vi "roboRIO Update Name Color.vi"(7 "FcdVI Ref":refnum<vi>, 8 "error in (no error)":errorcluster, 11 "Connector Name Ref":refnum<vi>) -> (0 "error out":errorcluster)   [LabVIEW 2021]
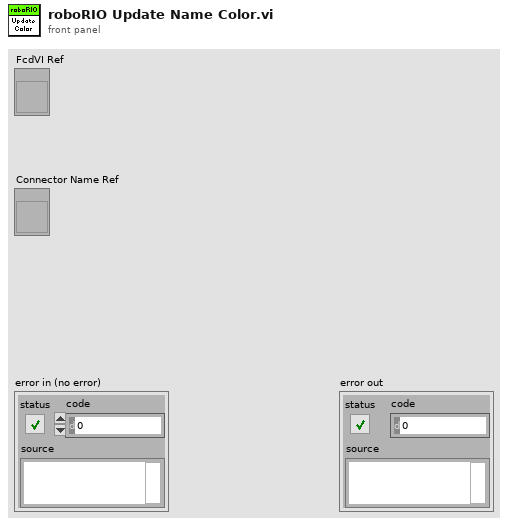
[diagram p1: front panel]
types:
  T1 = typedef "LVForegroundBackgroundColorsTypeDef.ctl" = cluster{"FG Color":u32, "BG Color":u32}
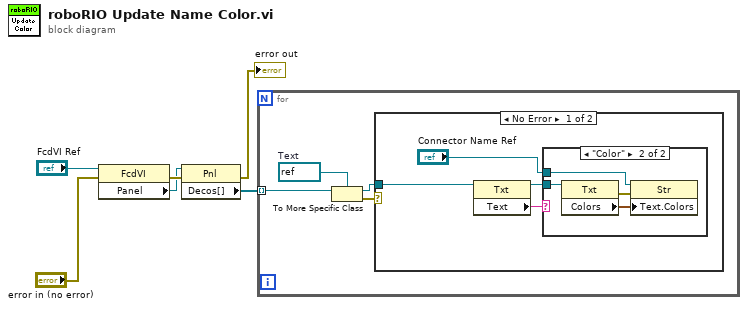
[diagram p0: block diagram]
diagram:
  n1 = property class="FcdVI"(reference="FcdVI Ref", error in="error in (no error)") -> (error out=w5:errorcluster, "Panel"=w4:refnum<vi>)  [unwired: 1 out]
  n2 = property class="Pnl"(reference=w4, error in=w5) -> (error out=→"error out":errorcluster, "Decos[]"=w3:refnum<vi>[])  [unwired: 1 out]
  n3 = for {
    tunnel: w3 -> [w10] mode=indexing
    w9 = refnum<vi> refnum  # Text
    n4 = To More Specific Class(target class=w9, reference=w10) -> (specific class reference=w7:refnum<vi>, error out=w8:errorcluster)  [unwired: 1 in]
    n5 = case shown="No Error" w8 {
      tunnel: w7 -> [w13 _]
      frame No Error {
        n6 = property class="Txt"(reference=w13) -> (reference out=w12:refnum<vi>, "Text"=w11:string)  [unwired: 1 in, 1 out]
        n7 = case shown="\"Color\"" w11 {
          tunnel: "Connector Name Ref" -> [_ w16]
          tunnel: w12 -> [_ w15]
          frame "False", Default {
          }
          frame "Color" {
            n8 = property class="Txt"(reference=w15) -> (error out=w18:errorcluster, "Colors"=w17:T1)  [unwired: 1 in, 1 out]
            n9 = property on="Property Node" class="Str"(reference=w16, error in=w18, "Text.Colors"=w17) -> ()  [unwired: 2 out]
          }
        }
      }
      frame Error {
      }
    }
  }
